vi "ECS Live Dumps.vi"(0 "Start Date and Time":string, 1 "End Date and Time":string, 2 "Device Name":string, 3 "Variable Name":string, 4 "Values":string[](array[string]), 5 "error constant":errorcluster) -> ()   [LabVIEW 2013]
panel:
  out "Waveform Graph":dbl[](graph)
  out "error constant 2":errorcluster
  in  "Multicolumn Listbox":i32(listbox)
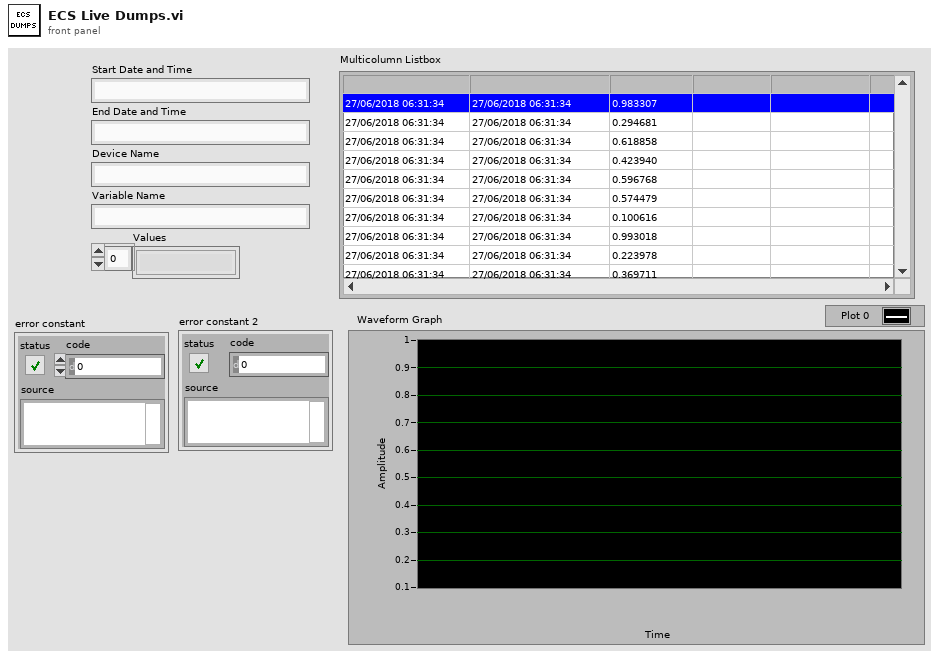
[diagram p1: front panel]
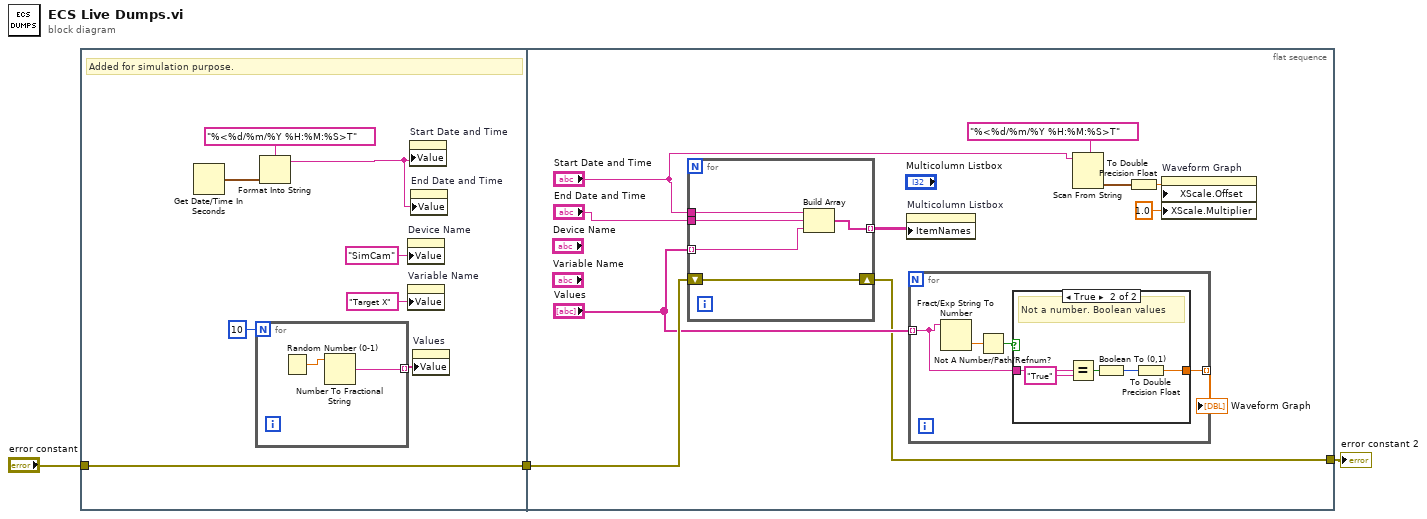
[diagram p0: block diagram]
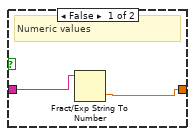
[diagram p2: hidden frame]
diagram:
  n1 = flat-sequence {
    tunnel: "error constant" -> [w7]
    tunnel: [w7] -> w2
    tunnel: w2 -> [w23]
    tunnel: [w14] -> w1
    frame #0 {
      # "Added for simulation purpose."
      n2 = Get Date/Time In Seconds() -> (seconds since 1Jan1904=w5:timestamp)
      n3 = for {
        N: 10 -> [_]
        tunnel: [w13] -> w10 mode=indexing
        n4 = Random Number (0-1)() -> (number: 0 to 1=w12:dbl)
        n5 = Number To Fractional String(number=w12) -> (F-format string=w13:string)  [unwired: 3 in]
      }
      n6 = Format Into String(format string="%<%d/%m/%Y %H:%M:%S>T", w5) -> (resulting string=w4:string)  [unwired: 2 in, 1 out]
      n7 = property on="Device Name" class="Str"("Value"="SimCam" ("Variable Name")) -> ()  [unwired: 2 in, 2 out]
      n8 = property on="Variable Name" class="Str"("Value"="Target X" ("Variable Name")) -> ()  [unwired: 2 in, 2 out]
      n9 = property on="Start Date and Time" class="Str"("Value"=w4) -> ()  [unwired: 2 in, 2 out]
      n10 = property on="End Date and Time" class="Str"("Value"=w4) -> ()  [unwired: 2 in, 2 out]
      n11 = property on="Values" class="Arr (strict)"("Value"=w10) -> ()  [unwired: 2 in, 2 out]
    }
    frame #1 {
      n12 = for {
        tunnel: "Start Date and Time" -> [w40]
        tunnel: "End Date and Time" -> [w39]
        tunnel: "Values" -> [w38] mode=indexing
        tunnel: [w37] -> w22 mode=indexing
        shift-right: [w36] -> w14
        shift-left: w23 -> [w36]
        n13 = Build Array(w40, w39, w38) -> (w37:string[])
      }
      n14 = property on="Multicolumn Listbox" class="MCListbox (strict)"("ItemNames"=w22) -> ()  [unwired: 2 in, 2 out]
      n15 = for {
        tunnel: "Values" -> [w28] mode=indexing
        tunnel: [w25] -> w20 mode=indexing
        n16 = Fract/Exp String To Number(string=w28) -> (number=w27:dbl)  [unwired: 3 in, 1 out]
        n17 = Not A Number/Path/Refnum?(number/path/refnum=w27) -> (NaN/Path/Refnum?=w26:bool)
        n18 = case shown="True" w26 {
          tunnel: w28 -> [w30 w35]
          tunnel: [w29 w31] -> w25
          frame False {
            # "Numeric values"
            n19 = Fract/Exp String To Number(string=w30) -> (number=w29:dbl)  [unwired: 3 in, 1 out]
          }
          frame True {
            # "Not a number. Boolean values"
            n20 = Equal?(x=w35, y="True") -> (x = y?=w33:bool)
            n21 = Boolean To (0,1)(Boolean=w33) -> (0, 1=w32:i16)
            n22 = To Double Precision Float(number=w32) -> (double precision float=w31:dbl)
          }
        }
      }
      "Waveform Graph" <- w20
      n23 = Scan From String(format string="%<%d/%m/%Y %H:%M:%S>T", input string="Start Date and Time") -> (output 1=w17:timestamp)  [unwired: 3 in, 3 out]
      n24 = To Double Precision Float(number=w17) -> (double precision float=w16:dbl)
      n25 = property on="Waveform Graph" class="WFGraph (strict)"("XScale.Offset"=w16, "XScale.Multiplier"=1.0 ("X Scale.Offset and Multiplier:Multiplier")) -> ()  [unwired: 2 in, 2 out]
    }
  }
  "error constant 2" <- w1
